vi "After Launch Init.vi"(8 "error in (no error)":errorcluster, 11 "Camera Simulator in":refnum<class "Camera Simulator.lvclass">) -> (0 "error out":errorcluster, 3 "Camera Simulator out":refnum<class "Camera Simulator.lvclass">)   [LabVIEW 2020, in "Camera Simulator.lvlib" / "Camera Simulator.lvclass"]
uses:
  Camera Simulator.lvclass
  C:/Program Files (x86)/National Instruments/LabVIEW 2020/vi.lib/ActorFramework/Actor/Actor.lvclass
  Camera Simulator Messages/Generate Image Msg/Generate Image Msg.lvclass
  C:/Program Files (x86)/National Instruments/LabVIEW 2020/vi.lib/ActorFramework/Message/Message.lvclass
  <vilib>/ActorFramework/Actor/Actor.lvclass/Actor.ctl
  <vilib>/ActorFramework/Message Enqueuer/Message Enqueuer.lvclass/Message Enqueuer.ctl
  Camera Simulator.lvclass/Camera Simulator.ctl
  <vilib>/numeric/Random Number (Range) I64.vi
  <vilib>/numeric/Random Number (Range) U64.vi
  <vilib>/numeric/sub_Random U32.vi
  <vilib>/ActorFramework/Message Enqueuer/Init from Existing Queue.vi
  Camera Actor/Camera Actor/Camera Actor.lvclass
  <vilib>/ActorFramework/Message Enqueuer/Message Enqueuer.lvclass
  <vilib>/ActorFramework/Actor/Actor.lvclass
  Camera Simulator.lvlib
panel:
  in  "Amplitude":i32=1000
  in  "Image X size":i32=1040
  in  "Center x":dbl=520.0 format="%#_13g"
  in  "Center y":dbl=520.0 format="%#_13g"
  in  "Image Y size":i32=1040
  in  "1/e HWidth":dbl=400.0 format="%#_13g"
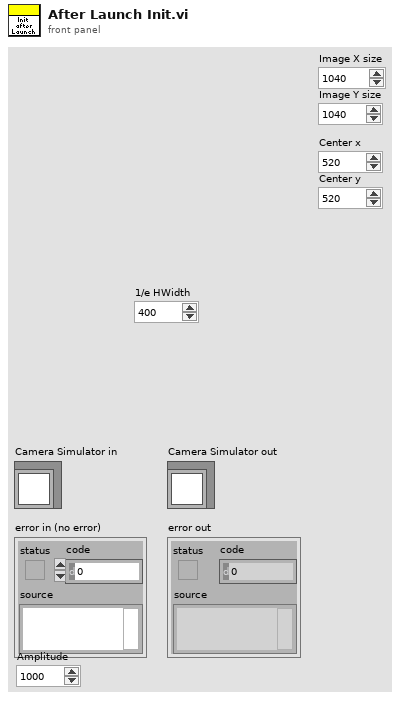
[diagram p1: front panel]
types:
  T1 = typedef "Image Type" = u32
  T2 = typedef "IMAQ Image.ctl" = refnum<image>
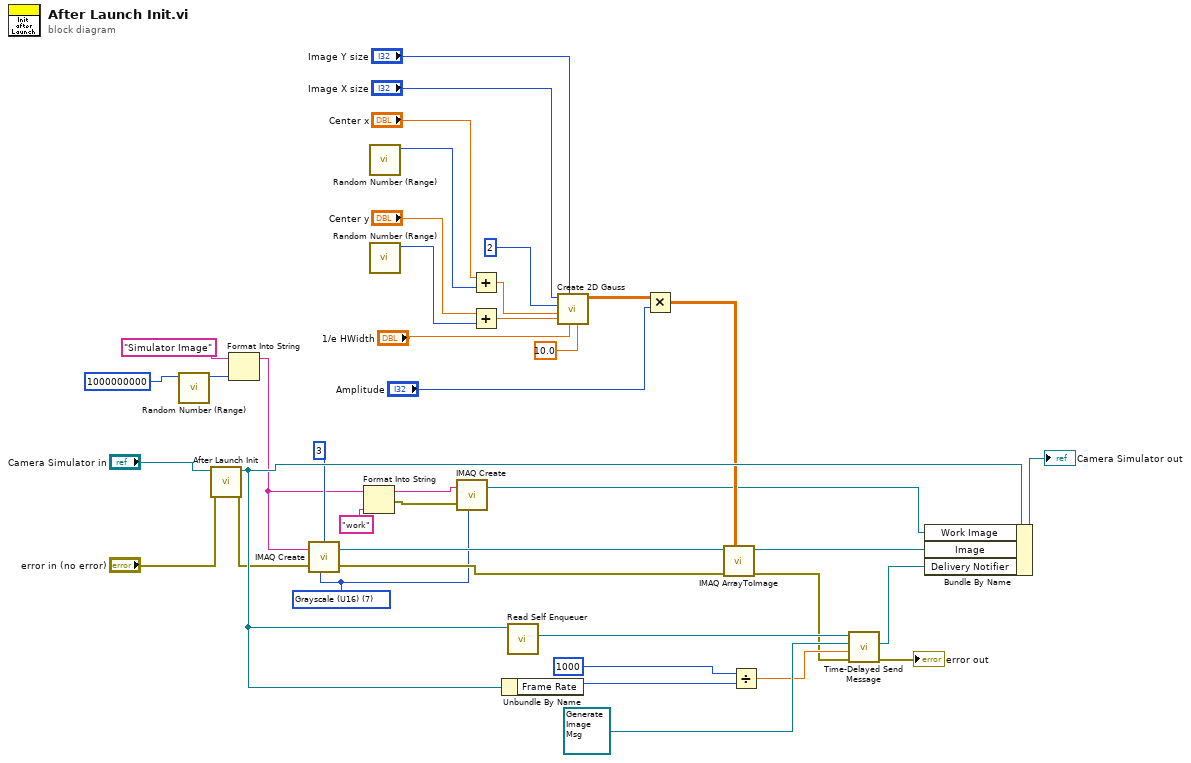
[diagram p0: block diagram]
diagram:
  w6 = T1 7 items=["Grayscale (U8)", "Grayscale (I16)", "Grayscale (SGL)", "Complex (CSG)", "RGB (U32)", "HSL (U32)", "RGB (U64)", "Grayscale (U16)"] ("Image Type")
  n1 = call-poly <vilib>:"Random Number (Range).vi"("upper bound (100)"=u64 1000000000) -> ("number"=w33:u64)  [unwired: 10 in]
  n2 = call-parent "After Launch Init.vi"("error in (no error)"="error in (no error)", "Camera Actor in"="Camera Simulator in") -> ("error out"=w36:errorcluster, "Camera Actor out"=w40:refnum<class "Camera Simulator.lvclass">)  [unwired: 8 in]
  n3 = Format Into String(initial string="Simulator Image" ("Image Name"), w33) -> (resulting string=w4:string)  [unwired: 2 in, 1 out]
  n4 = call "IMAQ Create"("Border Size"=3, "Image Name"=w4, "Image Type"=w6, "error in (no error)"=w36) -> ("New Image"=w13:T2, "error out"=w10:errorcluster)  [unwired: 1 in]
  n5 = Format Into String(initial string=w4, "work") -> (resulting string=w2:string, error out=w5:errorcluster)  [unwired: 2 in]
  n6 = call-poly <vilib>:"Random Number (Range).vi"() -> ("number"=w23:i64)  [unwired: 11 in]
  n7 = call-poly <vilib>:"Random Number (Range).vi"() -> ("number"=w21:i64)  [unwired: 11 in]
  n8 = call "IMAQ Create"("Image Name"=w2, "Image Type"=w6, "error in (no error)"=w5) -> ("New Image"=w1:T2)  [unwired: 2 in, 1 out]
  n9 = Add(x="Center x", y=w23) -> (x+y=w22:dbl)
  n10 = Add(x="Center y", y=w21) -> (x+y=w20:dbl)
  n11 = Unbundle By Name(w40) -> ("Frame Rate"=w30:u32)
  n12 = call <vilib>:"Read Self Enqueuer.vi"("Actor"=w40) -> ("Self Enqueuer"=w31:refnum<class "Message Enqueuer.lvclass">)  [unwired: 10 in]
  n13 = call "Create 2D Gauss.vi"("Rauschen %"=10.0, "1/e HWidth"="1/e HWidth", "Y size"="Image Y size", "mitte y"=w20, "mitte x"=w22, "Order"=2, "X size"="Image X size") -> ("2D Gauss"=w11:sgl[][])  [unwired: 3 in, 1 out]
  n14 = Multiply(x=w11, y="Amplitude") -> (x*y=w8:sgl[][])
  n15 = call "IMAQ ArrayToImage"("Image Pixels (U16)"=w8, "error in (no error)"=w10, "Image"=w13) -> ("error out"=w9:errorcluster, "Image Out"=w12:T2)  [unwired: 7 in]
  n16 = Divide(x=u32 1000, y=w30) -> (x/y=w28:dbl)
  n17 = call <vilib>:"Time-Delayed Send Message.vi"("error in (no error)"=w9, "Milliseconds To Wait"=w28, "Message"=refnum<class "Generate Image Msg.lvclass"> refnum ("Camera Simulator.lvlib:Generate Image Msg.lvclass"), "Message Enqueuer"=w31) -> ("error out"=→"error out":errorcluster, "Delivery Notifier"=w25:refnum<notifier>)  [unwired: 6 in]
  n18 = Bundle By Name(cluster=w40, "Work Image"=w1, "Image"=w12, "Delivery Notifier"=w25) -> (→"Camera Simulator out":refnum<class "Camera Simulator.lvclass">)
